vi "Auto-Write to Folder and file for pFC_YCC.vi"(0 "Current PD (mV)":dbl, 4 "Who's Data":enum16{"YCC", "PYW", "LCH", "YYH"}(ring), 5 "T=2D\nF=1D":bool=TRUE, 6 "2D data to be saved":dbl[][](array[numeric]) format="%0.2f", 7 "1D data to be saved":dbl[](array[numeric]) format="%0.2f", 8 "File name add to the end \n(height)":string="h300", 9 "Save?":bool) -> (2 "Save to File Name":string, 3 "Save to Path":path)   [LabVIEW 2014]
uses:
  <vilib>/Utility/file.llb/Write To Spreadsheet File (DBL).vi
panel:
  out "Folder name":string
  out "folder exists?":bool
  out "date/time string":string
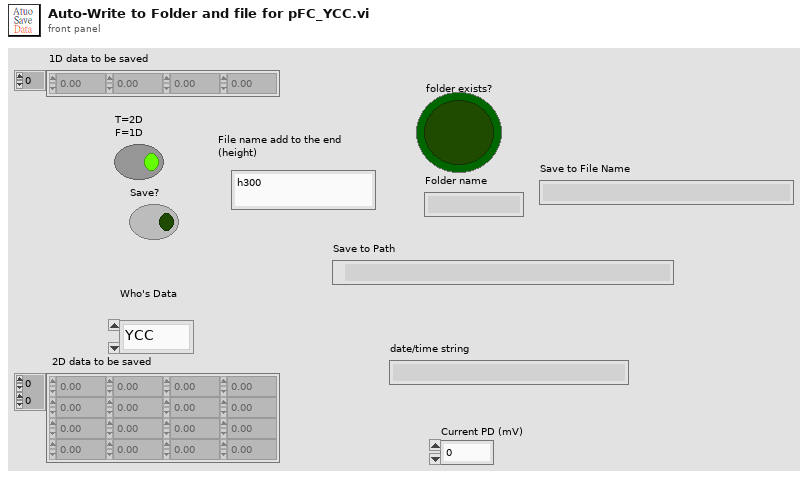
[diagram p1: front panel]
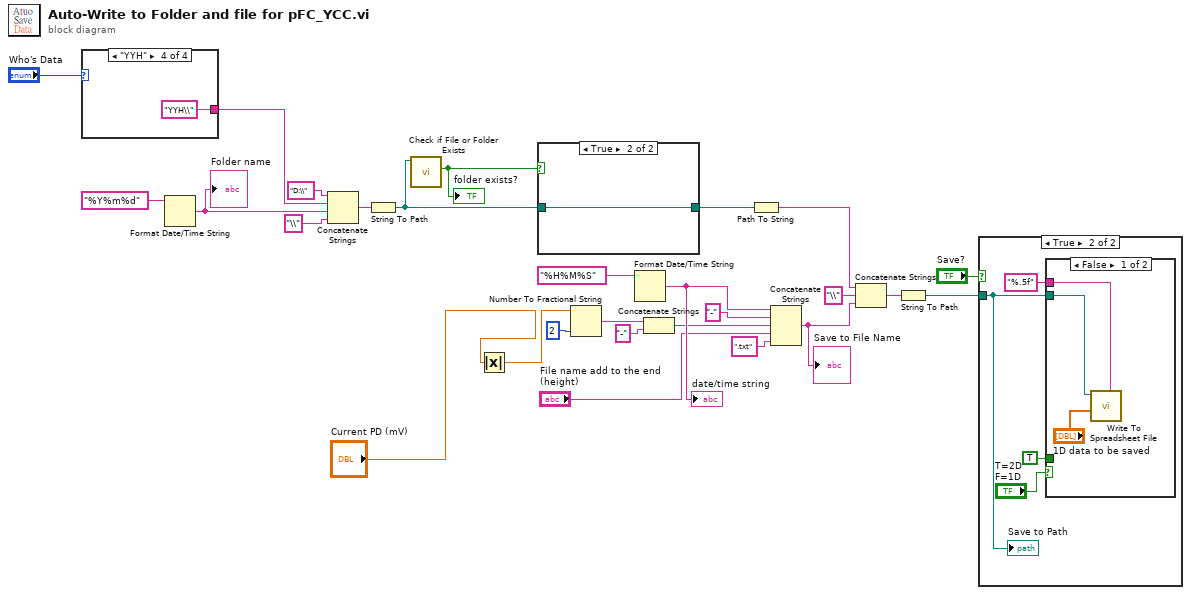
[diagram p0: block diagram]
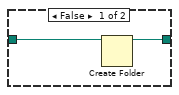
[diagram p2: hidden frame]
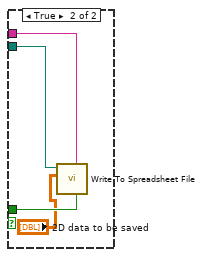
[diagram p4: hidden frame]
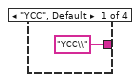
[diagram p5: hidden frame]
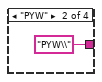
[diagram p6: hidden frame]
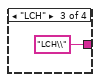
[diagram p7: hidden frame]
diagram:
  n1 = case shown="\"YYH\"" "Who's Data" {
    tunnel: ["YCC\\" ("string") "PYW\\" ("string") "LCH\\" ("string") "YYH\\" ("string")] -> w25
    frame "YCC", Default {
    }
    frame "PYW" {
    }
    frame "LCH" {
    }
    frame "YYH" {
    }
  }
  n2 = Format Date/Time String(time format string (%c)="%Y%m%d") -> (date/time string=w12:string)  [unwired: 2 in]
  "Folder name" <- w12
  n3 = Concatenate Strings("D:\\" ("string"), w25, w12, "\\" ("string")) -> (w24:string)
  n4 = String To Path(string=w24) -> (path=w15:path)
  n5 = call <vilib>:"Check if File or Folder Exists.vi"("path"=w15) -> ("file or folder exists?"=w14:bool)  [unwired: 8 in, 2 out]
  "folder exists?" <- w14
  n6 = Absolute Value(x="Current PD (mV)") -> (abs(x)=w2:dbl)
  n7 = case shown="True" w14 {
    tunnel: w15 -> [w33 w34]
    tunnel: [w32 w34] -> w20
    frame False {
      n8 = Create Folder(path (use dialog)=w33) -> (created path=w32:path)  [unwired: 2 in, 2 out]
    }
    frame True {
    }
  }
  n9 = Number To Fractional String(number=w2, precision (6)=i16 2) -> (F-format string=w6:string)  [unwired: 2 in]
  n10 = Format Date/Time String(time format string (%c)="%H%M%S") -> (date/time string=w10:string)  [unwired: 2 in]
  "date/time string" <- w10
  n11 = Concatenate Strings(w6, "-" ("string")) -> (w4:string)
  n12 = Path To String(path=w20) -> (string=w17:string)
  n13 = Concatenate Strings(w10, "-" ("string"), w4, "File name add to the end \n(height)", ".txt" ("string")) -> (w11:string)
  "Save to File Name" <- w11
  n14 = Concatenate Strings(w17, "\\" ("string"), w11) -> (w19:string)
  n15 = String To Path(string=w19) -> (path=w18:path)
  n16 = case shown="True" "Save?" {
    tunnel: w18 -> [_ w37]
    frame False {
    }
    frame True {
      n17 = case shown="False" "T=2D\nF=1D" {
        tunnel: TRUE ("transpose? (no:F)") -> [_ w45]
        tunnel: w37 -> [w40 w44]
        tunnel: "%.5f" ("format (%.3f)") -> [w41 w43]
        frame False {
          n18 = call-poly <vilib>:"Write To Spreadsheet File.vi"("format (%.3f)"=w41, "1D data"="1D data to be saved", "file path (dialog if empty)"=w40) -> ()  [unwired: 5 in, 1 out]
        }
        frame True {
          n19 = call-poly <vilib>:"Write To Spreadsheet File.vi"("transpose? (no:F)"=w45, "format (%.3f)"=w43, "2D data"="2D data to be saved", "file path (dialog if empty)"=w44) -> ()  [unwired: 4 in, 1 out]
        }
      }
      "Save to Path" <- w37
    }
  }
